vi "拉伸验证.vi"(0 "文件路径输入控件":path) -> (1 "弯曲刚度值":dbl, 2 "XY图":cluster{"Y":dbl[], "Y":dbl[]}[](graph))   [LabVIEW 2016]
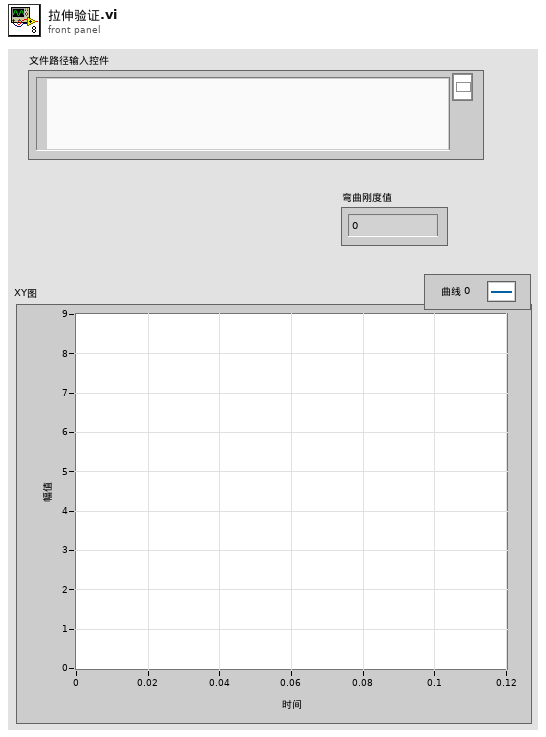
[diagram p1: front panel]
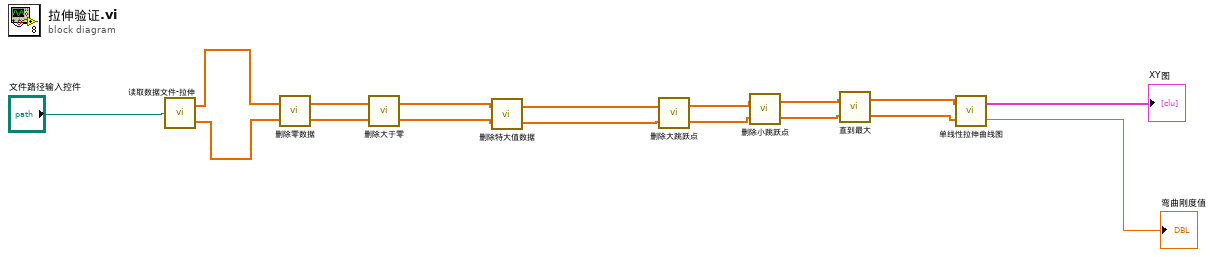
[diagram p0: block diagram]
diagram:
  n1 = call "读取数据文件-拉伸.vi"("文件路径（使用对话框）"="文件路径输入控件") -> ("第一列"=w16:dbl[], "第二列"=w15:dbl[])
  n2 = call "删除零数据.vi"("数组－数值 2"=w15, "数组－数值"=w16) -> ("第二列"=w13:dbl[], "第一列"=w14:dbl[])
  n3 = call "删除大于零.vi"("数组－数值 2"=w13, "数组－数值"=w14) -> ("第二列"=w7:dbl[], "第一列"=w8:dbl[])
  n4 = call "删除特大值数据.vi"("数组－数值 2"=w7, "数组－数值"=w8) -> ("数组 6"=w5:dbl[], "数组 5"=w6:dbl[])
  n5 = call "删除大跳跃点.vi"("数组－数值 2"=w5, "数组－数值"=w6) -> ("数组 6"=w11:dbl[], "数组 5"=w12:dbl[])
  n6 = call "删除小跳跃点.vi"("数组－数值 2"=w11, "数组－数值"=w12) -> ("第二列"=w9:dbl[], "第一列"=w10:dbl[])
  n7 = call "直到最大.vi"("数组－数值 2"=w9, "数组－数值"=w10) -> ("子数组 2"=w3:dbl[], "子数组"=w4:dbl[])
  n8 = call "单线性拉伸曲线图.vi"("数组－数值 2"=w3, "数组－数值"=w4) -> ("弯曲刚度值"=→"弯曲刚度值":dbl, "XY Graph"=→"XY图":cluster{"Y":dbl[], "Y":dbl[]}[])
